vi "字符串精度转换.vi"(7 "枚举":enum16{"小数位修约", "保留原始长度"}(ring), 9 "数组输入":string[](array[string]), 10 "数据精度":i32=6, 11 "输入字符串":string) -> (1 "数组输出":string[](array[string]), 3 "输出字符串":string)   [LabVIEW 2016, in "数据传输系统-02.lvlib"]
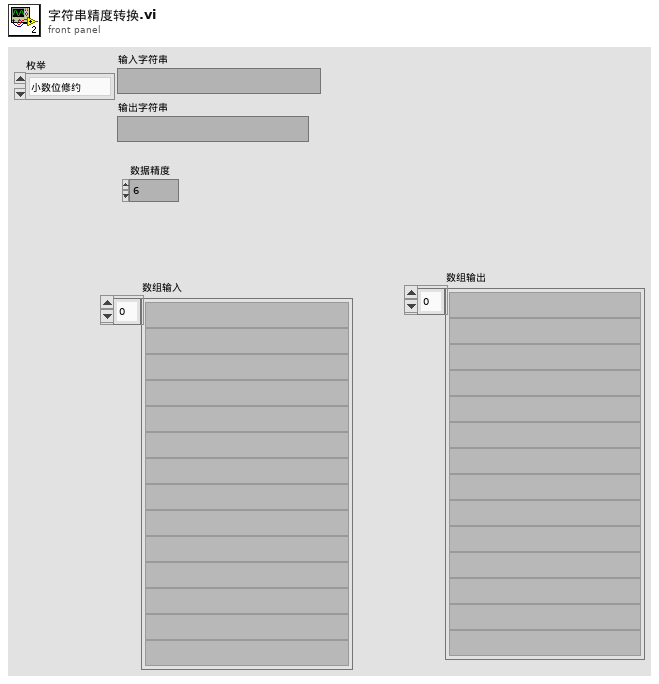
[diagram p1: front panel]
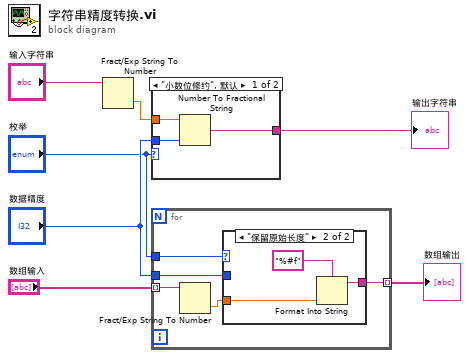
[diagram p0: block diagram]
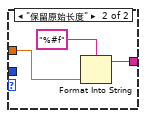
[diagram p2: hidden frame]
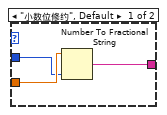
[diagram p3: hidden frame]
diagram:
  n1 = Fract/Exp String To Number(string="输入字符串") -> (number=w3:dbl)  [unwired: 3 in, 1 out]
  n2 = case shown="\"小数位修约\", 默认" "枚举" {
    tunnel: [w10 w11] -> w6
    tunnel: w3 -> [w9 w12]
    tunnel: "数据精度" -> [w8 _]
    frame "小数位修约", Default {
      n3 = Number To Fractional String(number=w9, precision (6)=w8) -> (F-format string=w10:string)  [unwired: 2 in]
    }
    frame "保留原始长度" {
      n4 = Format Into String(format string="%#f" ("格式字符串"), w12) -> (resulting string=w11:string)  [unwired: 2 in, 1 out]
    }
  }
  "输出字符串" <- w6
  n5 = for {
    tunnel: "数组输入" -> [w17] mode=indexing
    tunnel: [w16] -> w4 mode=indexing
    tunnel: "数据精度" -> [w15]
    tunnel: "枚举" -> [w14]
    n6 = Fract/Exp String To Number(string=w17) -> (number=w18:dbl)  [unwired: 3 in, 1 out]
    n7 = case shown="\"保留原始长度\"" w14 {
      tunnel: w18 -> [w21 w22]
      tunnel: [w20 w23] -> w16
      tunnel: w15 -> [w19 _]
      frame "小数位修约", Default {
        n8 = Number To Fractional String(number=w21, precision (6)=w19) -> (F-format string=w20:string)  [unwired: 2 in]
      }
      frame "保留原始长度" {
        n9 = Format Into String(format string="%#f" ("格式字符串"), w22) -> (resulting string=w23:string)  [unwired: 2 in, 1 out]
      }
    }
  }
  "数组输出" <- w4
